vi "Run Selected Tests.vi"(8 "error in (no error)":errorcluster, 10 "Tests":string[](array[string]), 11 "Execution UI In":refnum<class "Execution UI.lvclass">) -> (0 "error out":errorcluster, 3 "Execution UI Out":refnum<class "Execution UI.lvclass">)   [LabVIEW 2020, in "Execution UI.lvclass"]
uses:
  Execution UI.lvclass
  C:/git/astemes-lunit/source/Core/Result Observer/Result Observer.lvclass
  TypeDefs/Execution State.ctl
  Execution UI.lvclass/Execution UI.ctl
  Framework/Test Runner/Test Runner.lvclass
  Core/Runnable/Runnable.lvclass
  Result Model/Result Model.lvclass
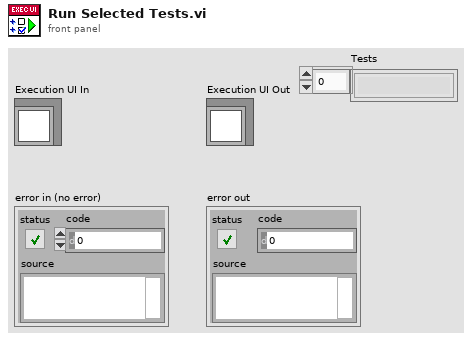
[diagram p1: front panel]
types:
  T1 = typedef "Execution UI.lvclass/Execution State.ctl" = enum16{"Idle", "Running"}
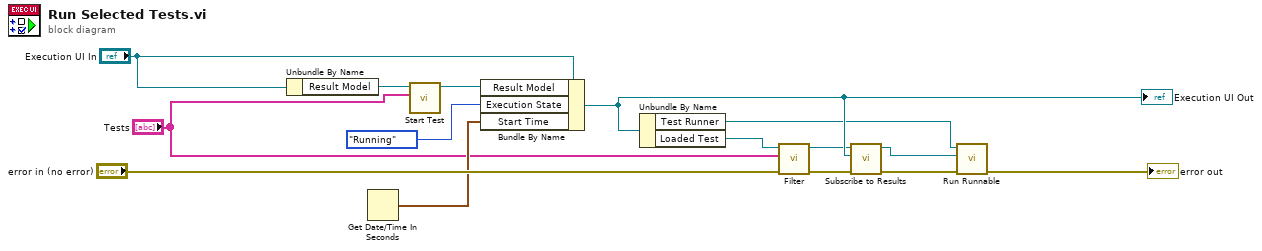
[diagram p0: block diagram]
diagram:
  n1 = Unbundle By Name("Execution UI In") -> ("Result Model"=w15:refnum<class "Result Model.lvclass">)
  n2 = Get Date/Time In Seconds() -> (seconds since 1Jan1904=w5:timestamp)
  n3 = call "Start Test.vi"("Tests"="Tests", "Result Model In"=w15) -> ("Result Model Out"=w14:refnum<class "Result Model.lvclass">)  [unwired: 9 in]
  n4 = Bundle By Name(cluster="Execution UI In", "Result Model"=w14, "Execution State"=Execution_State."Running", "Start Time"=w5) -> (w11:refnum<class "Execution UI.lvclass">)
  "Execution UI Out" <- w11
  n5 = Unbundle By Name(w11) -> ("Test Runner"=w3:refnum<class "Test Runner.lvclass">, "Loaded Test"=w9:refnum<class "Runnable.lvclass">)
  n6 = call-dynamic "Filter.vi"("error in (no error)"="error in (no error)", "Selected Runnables"="Tests", "Runnable In"=w9) -> ("error out"=w6:errorcluster, "Runnable Out"=w8:refnum<class "Runnable.lvclass">)  [unwired: 7 in]
  n7 = call-dynamic "Subscribe to Results.vi"("error in (no error)"=w6, "Result Observer"=w11, "Runnable In"=w8) -> ("error out"=w2:errorcluster, "Runnable Out"=w10:refnum<class "Runnable.lvclass">)  [unwired: 7 in]
  n8 = call-dynamic "Run Runnable.vi"("error in (no error)"=w2, "Runnable"=w10, "Test Runner In"=w3) -> ("error out"=→"error out":errorcluster)  [unwired: 8 in]
